vi "metadata.update_description.vi"(8 "error in":errorcluster, 9 "Description":string, 10 "Channel":refnum<class "Channel.lvclass">, 11 "Nominal Client in":refnum<class "Nominal Client.lvclass">) -> (0 "error out":errorcluster, 2 "Meta Data":T1, 3 "Nominal Client out":refnum<class "Nominal Client.lvclass">)   [LabVIEW 2020, in "Nominal Client.lvclass"]
uses:
  Nominal Client/Nominal Client.lvclass
  submodules/nominal-streaming-labview-ffi/lv_src/Channel/Channel.lvclass
  metadata.ctl
  Nominal Client/Nominal Client.lvclass/Nominal Client.ctl
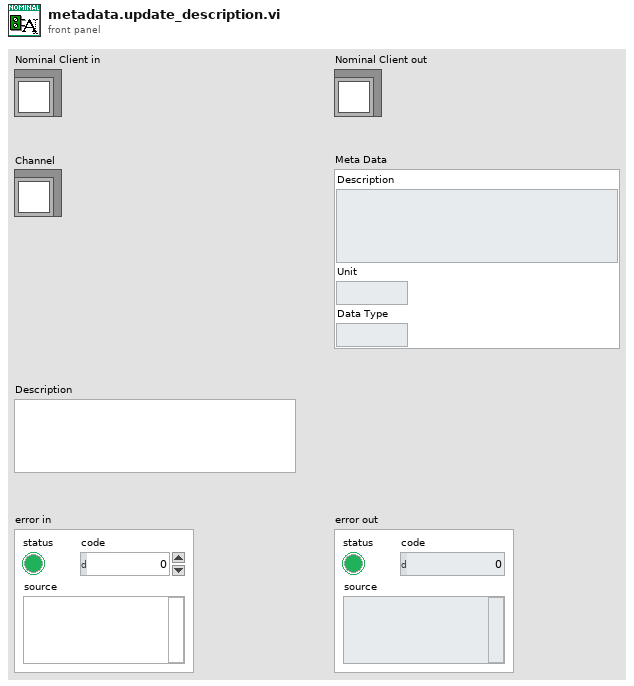
[diagram p1: front panel]
types:
  T1 = typedef "Nominal Client.lvclass/metadata.ctl" = cluster{"Description":string, "Unit":string, "Data Type":string}
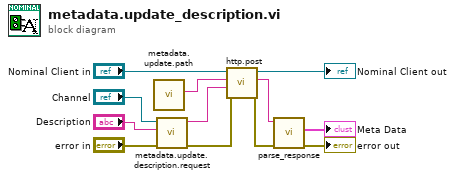
[diagram p0: block diagram]
diagram:
  n1 = call "metadata.update.path.vi"() -> ("path"=w6:string)  [unwired: 11 in]
  n2 = call "metadata.update.description.request.vi"("error in"="error in", "Description"="Description", "channel in"="Channel") -> ("error out"=w1:errorcluster, "JSON Payload"=w2:string)  [unwired: 7 in]
  n3 = call "http.post.vi"("error in"=w1, "Request body"=w2, "Path"=w6, "Nominal Client in"="Nominal Client in") -> ("error out"=w9:errorcluster, "Response"=w10:string, "Nominal Client out"=→"Nominal Client out":refnum<class "Nominal Client.lvclass">)  [unwired: 5 in]
  n4 = call "parse_response.vi"("error in"=w9, "Response"=w10) -> ("error out"=→"error out":errorcluster, "Meta Data"=→"Meta Data":T1)  [unwired: 8 in]
